vi "Example Callback - StateChanged Callback.vi"(4 "StateChanged":refnum<user-event>, 5 "Event Data":T1, 6 "Control Ref":refnum<k24>, 7 "Event Common Data":T2) -> ()   [LabVIEW 2010]
uses:
  C:/tf/play/labview/Tinkerforge.dll
  Tinkerforge.dll
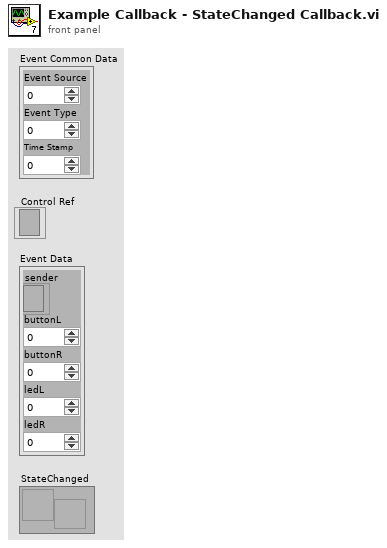
[diagram p1: front panel]
types:
  T1 = cluster{"sender":refnum<k24>, "buttonL":u8, "buttonR":u8, "ledL":u8, "ledR":u8}
  T2 = cluster{"Event Source":i32, "Event Type":u32, "Time Stamp":u32}
  T3 = cluster{"buttonL":u8, "buttonR":u8, "ledL":u8, "ledR":u8}
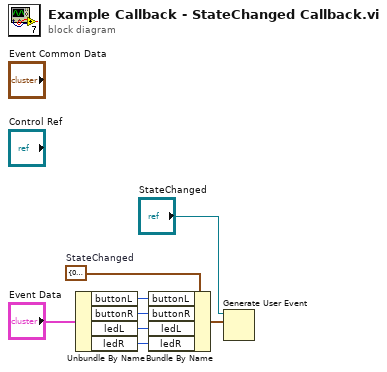
[diagram p0: block diagram]
diagram:
  w6 = T3 {"buttonL"=0, "buttonR"=0, "ledL"=0, "ledR"=0}  # StateChanged
  n1 = Unbundle By Name("Event Data") -> ("buttonL"=w4:u8, "buttonR"=w3:u8, "ledL"=w2:u8, "ledR"=w1:u8)
  n2 = Bundle By Name(cluster=w6, "buttonL"=w4, "buttonR"=w3, "ledL"=w2, "ledR"=w1) -> (w7:T3)
  n3 = Generate User Event(user event="StateChanged", event data cluster=w7) -> ()  [unwired: 1 in, 2 out]
